vi "Method_Const.vi"(4 "Value":u8, 5 "Value A":refnum<class "Abs_U8 Integer.lvclass">) -> (1 "Result":refnum<class "Abs_Boolean.lvclass">)   [LabVIEW 2021, in "Equal_U8.lvclass"]
uses:
  Equal_U8.lvclass
  Abs_Types/U8 Integer/Abs_U8 Integer.lvclass
  Abs_Types/Boolean/Abs_Boolean.lvclass
  C:/TSA/LV_Abstract/Source/Functions/Support/Compare/Two Term/U8/AbsComp_Two Term_U8.lvclass
  C:/Program Files (x86)/National Instruments/LabVIEW 2021/vi.lib/TSA/Abstract Data Classes/Abs_Types/Boolean/Abs_Boolean.lvclass
  Support/Compare/Two Term/U8/AbsComp_Two Term_U8.lvclass/AbsComp_Two Term_U8.ctl
  Support/Compare/Two Term/U8/Properties/Write Numeric A.vi
  Support/Compare/Two Term/U8/Properties/Write Numeric B.vi
  Constants/Support/U8/Const_U8.lvclass
  C:/Program Files (x86)/National Instruments/LabVIEW 2021/vi.lib/TSA/Abstract Data Classes/Abs_Types/Numeric/Abs_Numeric.lvclass
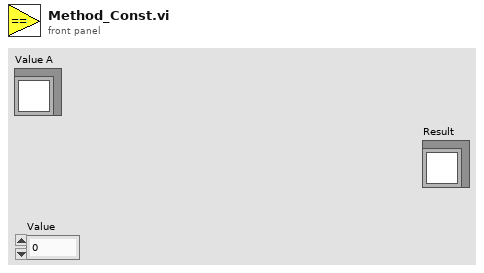
[diagram p1: front panel]
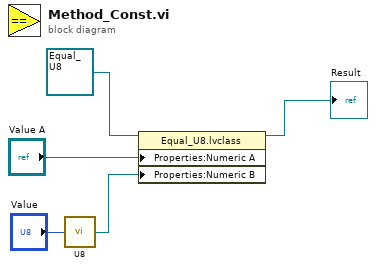
[diagram p0: block diagram]
diagram:
  n1 = call "U8.vi"("Value"="Value") -> ("Constant"=w2:refnum<class "Const_U8.lvclass">)  [unwired: 4 in]
  n2 = property class="Equal_U8.lvclass"(reference=refnum<class "Equal_U8.lvclass"> refnum ("Greater 0_U64.lvclass"), "Properties:Numeric A"="Value A", "Properties:Numeric B"=w2) -> (reference out=→"Result":refnum<class "Equal_U8.lvclass">)  [unwired: 1 in, 1 out]
